vi "Prepare.vi"(8 "error in":errorcluster, 10 "Iterator Settings":T1={"Prepare timeout (ms)"=200, "Iterate timeout (ms)"=50, "Conclude timeout (ms)"=200, "Iterate period (ms)"=200, "Number of iterations"=5, "Time before stop (ms)"=5, "Active Stop Conditions"={"Number of Iterations"=FALSE, "Time Elapsed"=FALSE, "Iteration Result"=FALSE}, "Prepare Msg"=refnum, "Iterate Msg"=refnum, "Conclude Msg"=refnum, "Iterations End Report"=refnum, "Message Priority (Normal)"=enum."Normal"}, 11 "Iterator Actor in":refnum<class "Iterator NR Actor.lvclass">) -> (0 "error out":errorcluster, 2 "Reply":bool, 3 "Iterator Actor out":refnum<class "Iterator NR Actor.lvclass">)   [LabVIEW 2023, in "Iterator Actor.lvlib" / "Iterator NR Actor.lvclass"]
doc: "Calls the Prepare method of the Client and receives its responce."
uses:
  Iterator NR Actor.lvclass
  Abstract Iterator Actor/Iterator Settings.ctl
  Abstract Iterator Actor Messages/Iterator Report Iterations End Msg/Iterator Report Iterations End Msg.lvclass
  <vilib>/ActorFramework/Message/Message.lvclass
  Abstract Iterator Actor/Active Stop Conditions.ctl
  <vilib>/ActorFramework/Message Enqueuer/Message Priority.ctl
  C:/Projects/Iterator Actor/Abstract Iterator Actor/Abstract Iterator Actor.lvclass
  C:/Program Files/National Instruments/LabVIEW 2023/vi.lib/ActorFramework/Actor/Actor.lvclass
  Abstract Iterator Actor/Abstract Iterator Actor.lvclass/Abstract Iterator Actor.ctl
  <vilib>/ActorFramework/Actor/Actor.lvclass/Actor.ctl
  Iterator NR Actor.lvclass/Iterator NR Actor.ctl
  <vilib>/ActorFramework/Batch Msg/Batch Msg.lvclass/Batch Msg.ctl
  <vilib>/ActorFramework/Message Enqueuer/Message Enqueuer.lvclass/Message Enqueuer.ctl
  Abstract Iterator Actor/Read Stop Iterate Notifier.vi
  <vilib>/ActorFramework/Actor/Read Caller Enqueuer.vi
  <vilib>/ActorFramework/Batch Msg/Send Batch.vi
  <vilib>/ActorFramework/Message Enqueuer/Enqueue.vi
  Iterator NR Actor Messages/Request Iteration Notification Msg/Request Iteration Notification Msg.lvclass
  C:/Program Files/National Instruments/LabVIEW 2023/vi.lib/ActorFramework/Message/Message.lvclass
  <vilib>/ActorFramework/Batch Msg/Batch Msg.lvclass
  <userlib>/_OpenG.lib/lvdata/lvdata.llb/LVOOP Is Same Or Descendant Class__ogtk.vi
  Abstract Iterator Actor/Read Settings.vi
  <vilib>/ActorFramework/Message Priority Queue/Priority Enqueue.vi
  <vilib>/Utility/error.llb/Error Cluster From Error Code.vi
  Iterator NR Actor Messages/Abstract Iteration Msg/Abstract Iteration Msg.lvclass
  <vilib>/ErrorRing/Error Ring.xnode
  Abstract Iterator Actor/Abstract Iterator Actor.lvclass
  <vilib>/ActorFramework/Message Enqueuer/Message Enqueuer.lvclass
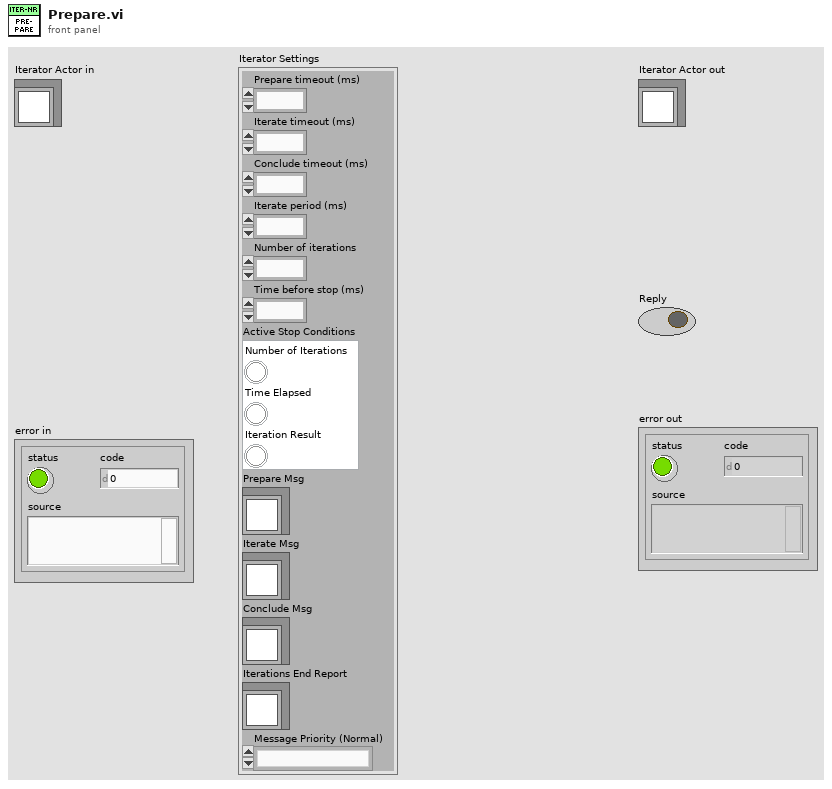
[diagram p1: front panel]
types:
  T1 = typedef "Iterator Actor.lvlib/Abstract Iterator Actor.lvclass/Iterator Settings.ctl" = cluster{"Prepare timeout (ms)":i32, "Iterate timeout (ms)":i32, "Conclude timeout (ms)":i32, "Iterate period (ms)":i32, "Number of iterations":i32, "Time before stop (ms)":i32, "Active Stop Conditions":T2, "Prepare Msg":refnum<class "Message.lvclass">, "Iterate Msg":refnum<class "Message.lvclass">, "Conclude Msg":refnum<class "Message.lvclass">, "Iterations End Report":refnum<class "Iterator Report Iterations End Msg.lvclass">, "Message Priority (Normal)":T3}
  T2 = typedef "Iterator Actor.lvlib/Abstract Iterator Actor.lvclass/Active Stop Conditions.ctl" = cluster{"Number of Iterations":bool, "Time Elapsed":bool, "Iteration Result":bool}
  T3 = typedef "Actor Framework.lvlib/Message Enqueuer.lvclass/Message Priority.ctl" = enum16{"Low", "Normal", "High"}
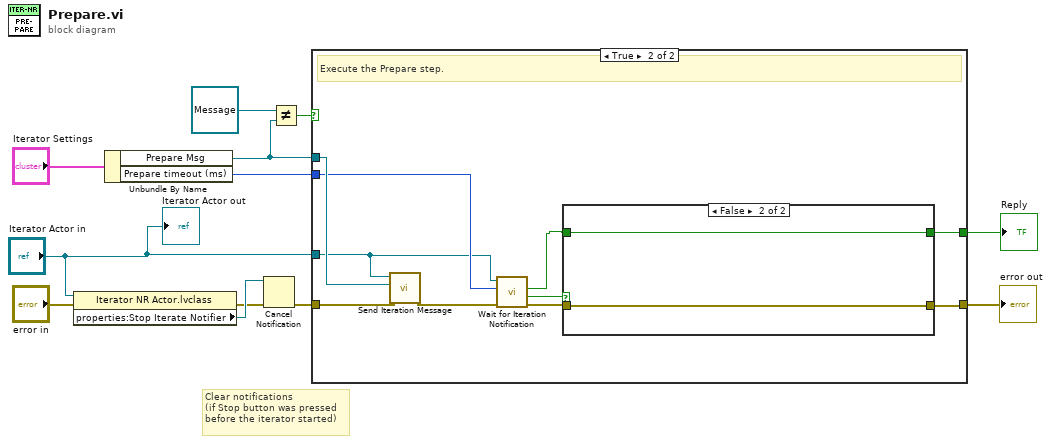
[diagram p0: block diagram]
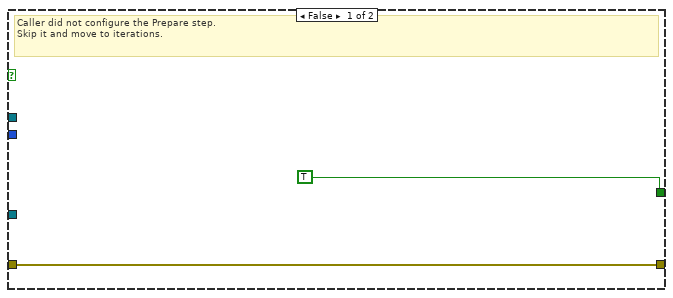
[diagram p2: hidden frame]
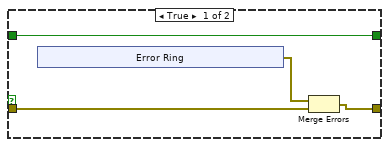
[diagram p3: hidden frame]
diagram:
  # "Clear notifications\n(if Stop button was pressed\nbefore the iterator started)"
  n1 = property class="Iterator NR Actor.lvclass"(reference="Iterator Actor in", error in="error in") -> (error out=w1:errorcluster, "properties:Stop Iterate Notifier"=w3:refnum<notifier>)  [unwired: 1 out]
  n2 = Unbundle By Name("Iterator Settings") -> ("Prepare Msg"=w5:refnum<class "Message.lvclass">, "Prepare timeout (ms)"=w12:i32)
  n3 = Cancel Notification(0:w3, 3:w1) -> (11:w9:errorcluster)  [unwired: 2 out]
  n4 = Not Equal?(x=refnum<class "Message.lvclass"> refnum ("Prepare Msg"), y=w5) -> (x != y?=w8:bool)
  n5 = case shown="True" w8 {
    tunnel: w12 -> [_ w21]
    tunnel: w5 -> [_ w24]
    tunnel: [TRUE w15] -> w7
    tunnel: [w14 w19] -> w10
    tunnel: w9 -> [w14 w23]
    tunnel: "Iterator Actor in" -> [_ w20]
    frame False {
      # "Caller did not configure the Prepare step.\nSkip it and move to iterations."
    }
    frame True {
      # "Execute the Prepare step."
      n6 = call "Send Iteration Message.vi"("error in (no error)"=w23, "Iteration Msg"=w24, "Iterator NR Actor in"=w20) -> ("error out"=w22:errorcluster)  [unwired: 8 in]
      n7 = call "Wait for Iteration Notification.vi"("error in (no error)"=w22, "timeout in ms (-1)"=w21, "Iterator NR Actor in"=w20) -> ("error out"=w18:errorcluster, "timed out?"=w17:bool, "Iterate?"=w16:bool)  [unwired: 5 in, 1 out]
      n8 = case shown="False" w17 {
        tunnel: w18 -> [w28 w34]
        tunnel: [w27 w34] -> w19
        tunnel: w16 -> [w25 w33]
        tunnel: [w25 w33] -> w15
        frame True {
          n9 = xnode "Error Ring"() -> ("error out"=w26:errorcluster)
          n10 = Merge Errors(w26, w28) -> (w27:errorcluster)
        }
        frame False {
        }
      }
    }
  }
  "Reply" <- w7
  "error out" <- w10
  "Iterator Actor out" <- "Iterator Actor in"
